vi "Get Window Bounds.vi"(7 "hWnd":u64) -> (8 "Window Bounds":i32[](array[numeric]))   [LabVIEW 2020]
uses:
  GETWINDOWBOUNDS.dll
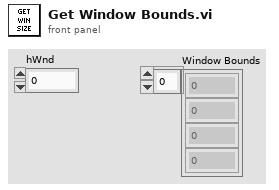
[diagram p1: front panel]
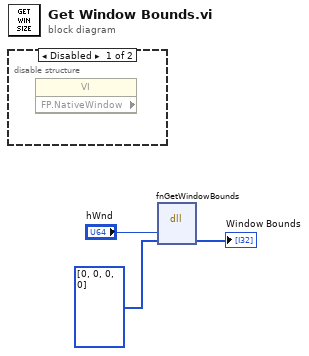
[diagram p0: block diagram]
diagram:
  n1 = disable-structure shown="Disabled" {
    frame Disabled {
      n2 = property class="VI" props=["FP.NativeWindow"]() -> ()  [unwired: 2 in, 3 out]
    }
    frame Enabled {
    }
  }
  n3 = dll-call lib="F:/OneDrive - University of Cambridge/Documents/Microscope-Control/Tools/Get Window Bounds/GETWINDOWBOUNDS.dll" fn="fnGetWindowBounds"("hWnd"="hWnd", "Input"=i32[] [0, 0, 0, 0]) -> ("Input"=→"Window Bounds":i32[])  [unwired: 5 in, 2 out]
